vi "MegaVIEW_v_0_0_2.vi"() -> ()   [LabVIEW 2016]
uses:
  <vilib>/Platform/TimedLoop/XDataNode/timing_clust.ctl
  <vilib>/Platform/TimedLoop/XDataNode/nitl_modes.ctl
  <vilib>/Platform/TimedLoop/XDataNode/wakeup.ctl
  <instrlib>/Lake Shore 425/Public/Data/Field Data (Single Reading).vi
  <vilib>/platform/TimedLoop/XDataNode/XDataNode.xnode
  <instrlib>/Lake Shore 425/Lake Shore 425.lvlib
  <vilib>/Platform/TimedLoop/XDataNode/XDNodeRunTimeDep.lvlib
panel:
  out "Numeric":i32
  in  "Position":dbl
  in  "Y Axis":i32(ring) items=["Time", "Position", "Gaussmeter 1", "Gaussmeter 2", "Gaussmeter 3", "Multimeter", "Temp. Monitor"]
  in  "X Axis":i32(ring) items=["Time", "Position", "Gaussmeter 1", "Gaussmeter 2", "Gaussmeter 3", "Multimeter", "Temp. Monitor"]
  out "XY Graph":cluster{dbl[], dbl[]}[](graph)
  in  "Seconds":dbl
  in  "Minutes":dbl
  in  "Hours":dbl
  out "Gaussmeter 3 Chart":dbl(graph)
  out "Gaussmeter 2 Chart":dbl(graph)
  out "Gaussmeter 1 Chart":dbl(graph)
  in  "Gaussmeter 3":bool
  out "Probe Field \nCompensation On 3":bool
  out "Probe Sensitivity 3":dbl=0.001 format="%^.3e"
  out "Probe Serial Number 3":string
  out "Probe Type  3":u16(ring)=40 items=["High Sensitivity"=40, "High Stability"=41, "Ultra-High Sensitivity"=42, "User Programmable Cable / High Sensitivity Probe"=50, "User Programmable Cable / High Stability Probe"=51, "User Programmable Cable / Ultra-High Sensitivity Probe"=52]
  out "Gaussmeter 3 Error":errorcluster
  in  "VISA Gaussmeter 3":refnum<visa-resource-name>
  in  "Gaussmeter 2":bool
  in  "Gaussmeter 1":bool
  in  "stop":bool
  out "Output File Path":path
  in  "Output Folder Path":path
  out "Output File Name":string
  in  "Period [s]":dbl format="%#_3g"
  out "Probe Field \nCompensation On 2":bool
  out "Probe Sensitivity 2":dbl=0.001 format="%^.3e"
  out "Probe Serial Number 2":string
  out "Probe Type  2":u16(ring)=40 items=["High Sensitivity"=40, "High Stability"=41, "Ultra-High Sensitivity"=42, "User Programmable Cable / High Sensitivity Probe"=50, "User Programmable Cable / High Stability Probe"=51, "User Programmable Cable / Ultra-High Sensitivity Probe"=52]
  out "Probe Field \nCompensation On 1":bool
  out "Probe Sensitivity 1":dbl=0.001 format="%^.3e"
  out "Probe Serial Number 1":string
  out "Probe Type 1":u16(ring)=40 items=["High Sensitivity"=40, "High Stability"=41, "Ultra-High Sensitivity"=42, "User Programmable Cable / High Sensitivity Probe"=50, "User Programmable Cable / High Stability Probe"=51, "User Programmable Cable / Ultra-High Sensitivity Probe"=52]
  out "Gaussmeter 2 Error":errorcluster
  out "Gaussmeter 1 Error":errorcluster
  in  "VISA Gaussmeter 2":refnum<visa-resource-name>
  in  "VISA Gaussmeter 1":refnum<visa-resource-name>
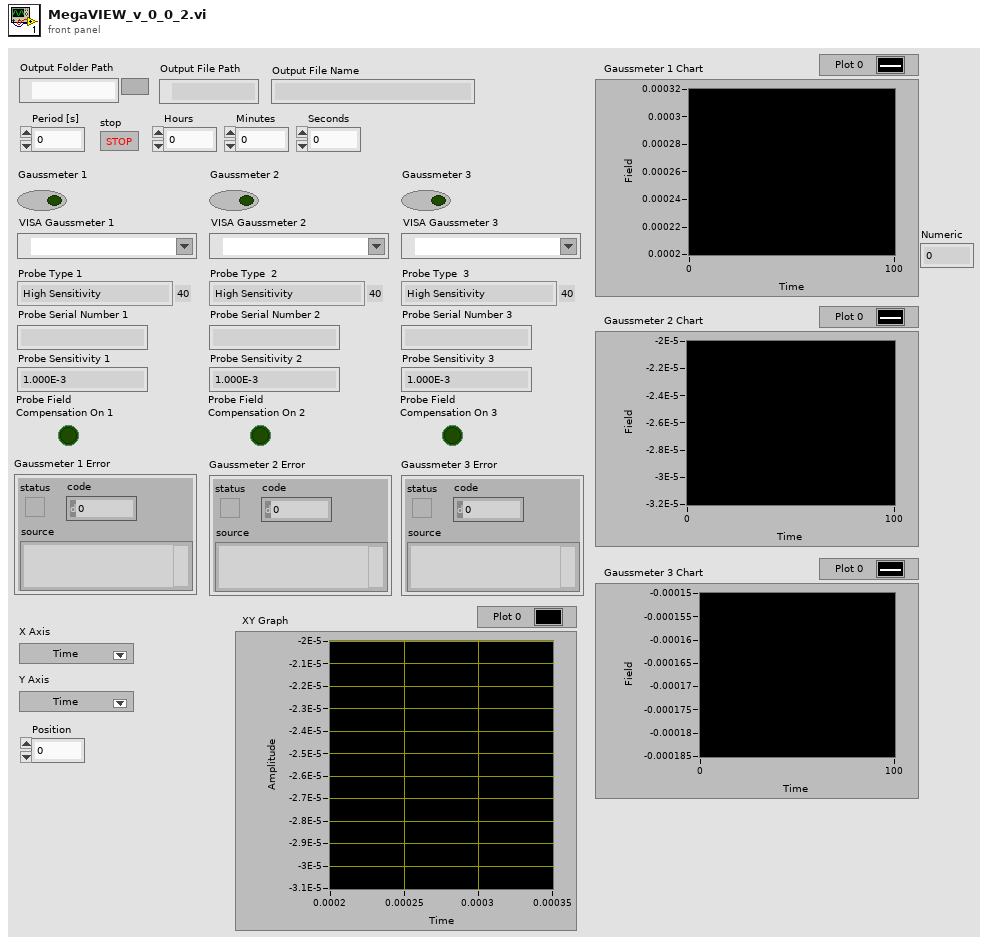
[diagram p1: front panel]
types:
  T1 = enum16{"open", "replace", "create", "open or create", "replace or create", "replace or create with confirmation"}
  T2 = typedef "XDNodeRunTimeDep.lvlib/timing_clust.ctl" = cluster{"Expected End [f-1]":u64, "Actual End [f-1]":u64, "Finished Late? [f-1]":bool, "Expected End [i-1]":u64, "Actual End [i-1]":u64, "Finished Late? [i-1]":bool, "Expected Start [i]":u64, "Actual Start [i]":u64, "Expected Start [f]":u64, "Actual Start [f]":u64, "Source Name":string, "Structure Name":string, "Period":i64, "Deadline":i64, "Offset":i64, "Start":i64, "Priority":i32, "Timeout":i32, "Mode":T3, "Wakeup Reason":T4, "Error":errorcluster, "Source Type":string, "Secondary Source Type":string, "Global End Time":u64, "Global Start Time":u64, "Frame Duration":u64, "Iteration Duration":u64, "Assigned CPU":i32, "I/O Scan Engine Mode":u32}
  T3 = typedef "XDNodeRunTimeDep.lvlib/nitl_modes.ctl" = enum32{"No Change", "Process missed periods, maintain original phase", "Discard missed periods, maintain original phase", "Process missed periods, ignore original phase", "Discard missed periods, ignore original phase"}
  T4 = typedef "XDNodeRunTimeDep.lvlib/wakeup.ctl" = enum32{"Normal", "Aborted", "Asynchronous wakeup", "Timing source error", "Timed loop error", "Timeout"}
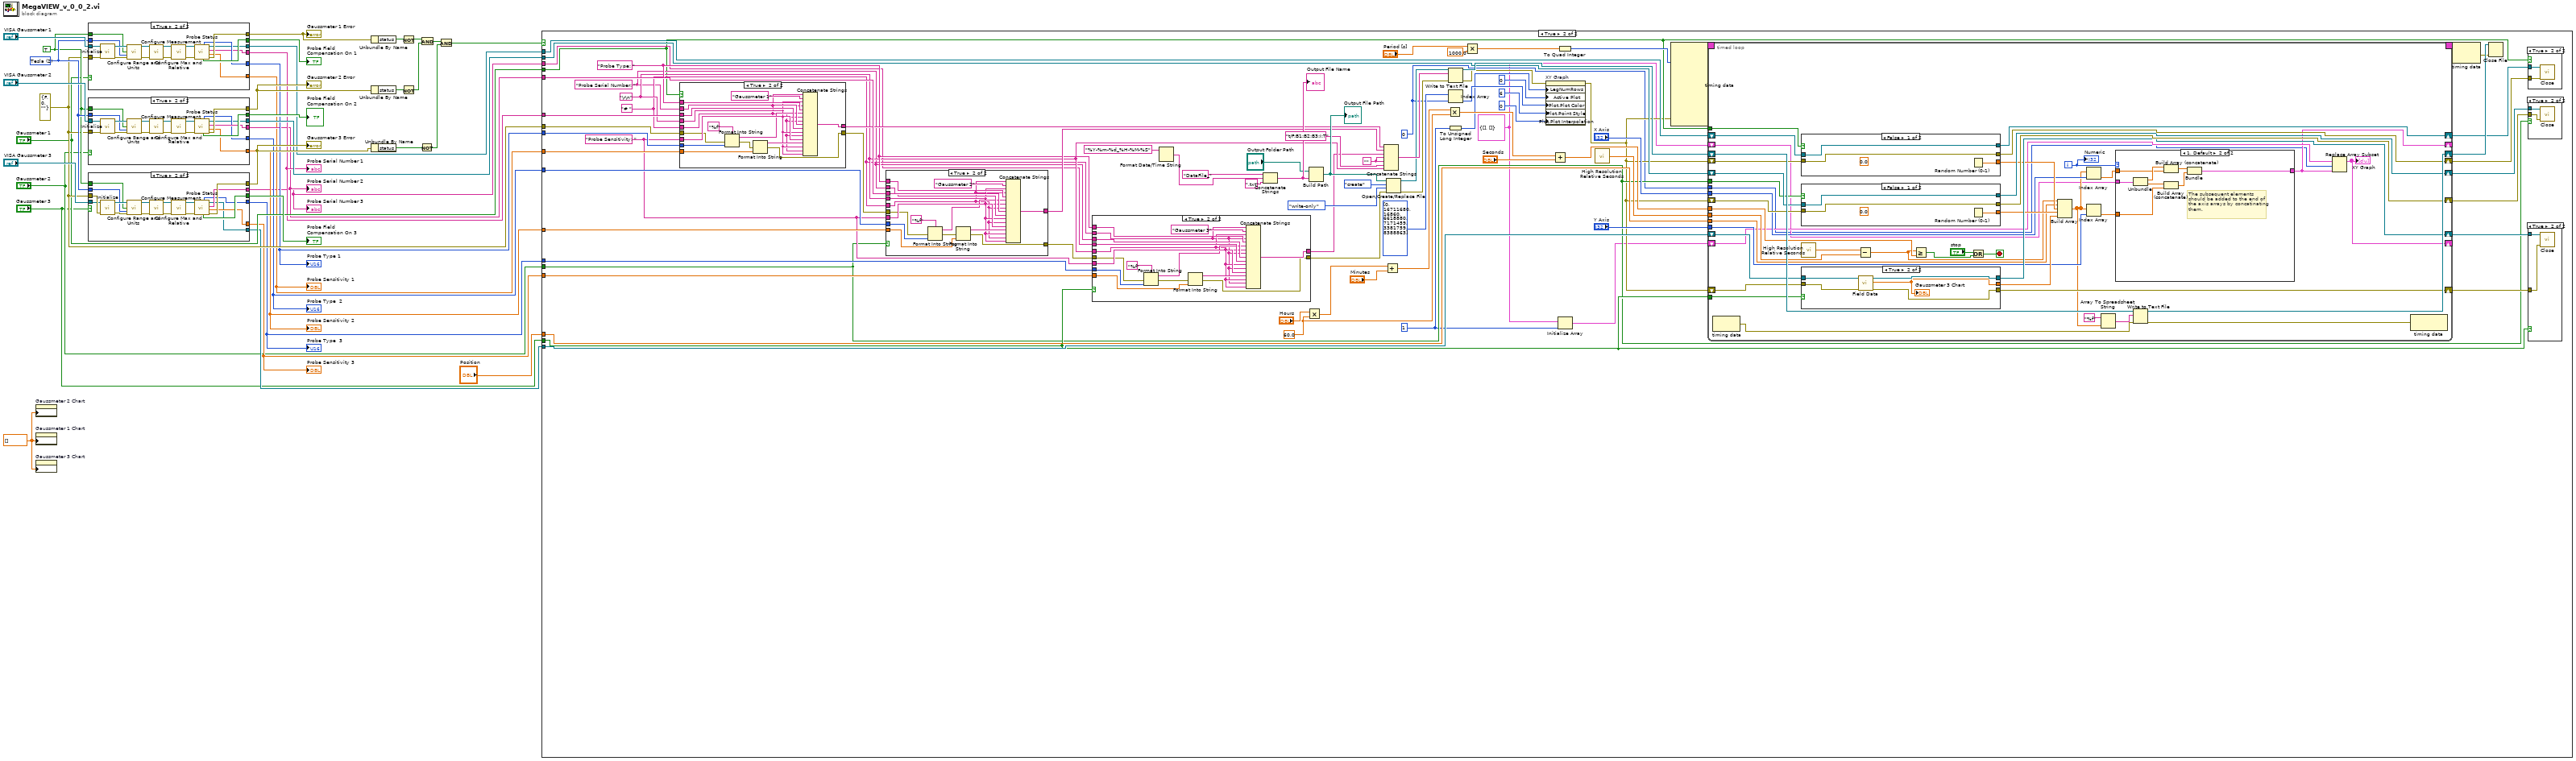
[diagram p0: block diagram]
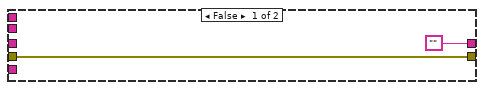
[diagram p6: hidden frame]
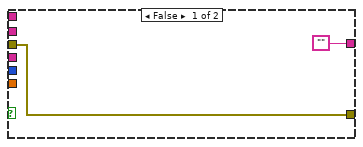
[diagram p7: hidden frame]
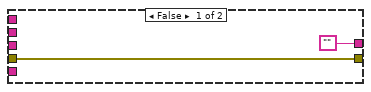
[diagram p8: hidden frame]
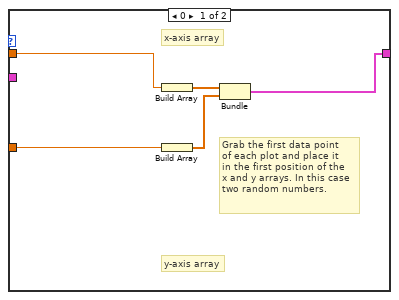
[diagram p9: hidden frame]
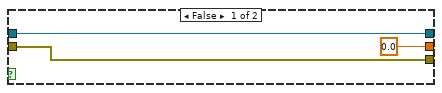
[diagram p10: hidden frame]
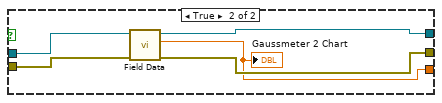
[diagram p11: hidden frame]
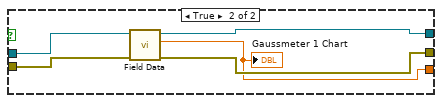
[diagram p12: hidden frame]
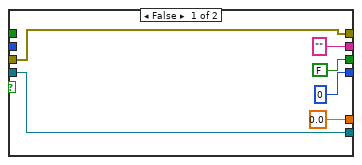
[diagram p13: hidden frame]
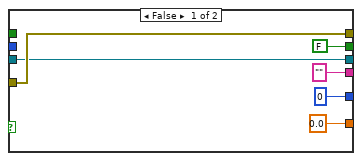
[diagram p14: hidden frame]
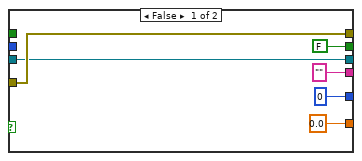
[diagram p15: hidden frame]
diagram:
  w15 = dbl[] [] ("History Data")
  w35 = u16 2 items=["Gauss"=1, "Tesla"=2, "Oersted"=3, "Amp/meter"=4] ("Field Units (1:Gauss)")
  w34 = TRUE ("Auto Range (F: Off)")
  w18 = errorcluster {"status"=FALSE, "code"=0, "source"=""} ("error in (no error)")
  n1 = property on="Gaussmeter 2 Chart" class="WFChart (strict)"("History Data"=w15) -> ()  [unwired: 2 in, 2 out]
  n2 = property on="Gaussmeter 1 Chart" class="WFChart (strict)"("History Data"=w15) -> ()  [unwired: 2 in, 2 out]
  n3 = property on="Gaussmeter 3 Chart" class="WFChart (strict)"("History Data"=w15) -> ()  [unwired: 2 in, 2 out]
  n4 = case shown="True" "Gaussmeter 1" {
    tunnel: "VISA Gaussmeter 1" -> [w38 w61]
    tunnel: w35 -> [_ w58]
    tunnel: w34 -> [_ w57]
    tunnel: w18 -> [w43 w56]
    tunnel: [w43 w55] -> w31
    tunnel: [FALSE w54] -> w19
    tunnel: [u16 0 ("Probe Type") w53] -> w12
    tunnel: ["" ("Probe Serial Number") w52] -> w11
    tunnel: [0.0 ("Probe Sensitivity") w51] -> w8
    tunnel: [w38 w44] -> w16
    frame False {
    }
    frame True {
      n5 = call <instrlib>:"Initialize.vi"("error in (no error)"=w56, "VISA resource name"=w61) -> ("error out"=w59:errorcluster, "VISA resource name out"=w60:refnum<visa-resource-name>)  [unwired: 8 in]
      n6 = call <instrlib>:"Configure Range and Units.vi"("VISA resource name"=w60, "Auto Range (F: Off)"=w57, "Field Units (1:Gauss)"=w58, "error in (no error)"=w59) -> ("VISA resource name out"=w50:refnum<visa-resource-name>, "error out"=w49:errorcluster)  [unwired: 10 in]
      n7 = call <instrlib>:"Configure Measurement.vi"("VISA resource name"=w50, "error in (no error)"=w49) -> ("VISA resource name out"=w46:refnum<visa-resource-name>, "error out"=w47:errorcluster)  [unwired: 12 in]
      n8 = call <instrlib>:"Configure Max and Relative.vi"("VISA resource name"=w46, "error in (no error)"=w47) -> ("VISA resource name out"=w45:refnum<visa-resource-name>, "error out"=w48:errorcluster)  [unwired: 12 in]
      n9 = call <instrlib>:"Probe Status.vi"("error in (no error)"=w48, "VISA resource name"=w45) -> ("error out"=w55:errorcluster, "Probe Sensitivity"=w51:dbl, "Probe Serial Number"=w52:string, "VISA resource name out"=w44:refnum<visa-resource-name>, "Probe Field \nCompensation On"=w54:bool, "Probe Type"=w53:u16)  [unwired: 4 in]
    }
  }
  "Gaussmeter 1 Error" <- w31
  "Probe Field \nCompensation On 1" <- w19
  "Probe Serial Number 1" <- w11
  "Probe Sensitivity 1" <- w8
  "Probe Type 1" <- w12
  n10 = case shown="True" "Gaussmeter 2" {
    tunnel: "VISA Gaussmeter 2" -> [w62 w85]
    tunnel: w35 -> [_ w82]
    tunnel: w34 -> [_ w81]
    tunnel: w18 -> [w67 w80]
    tunnel: [w67 w79] -> w33
    tunnel: [FALSE w78] -> w21
    tunnel: [0.0 ("Probe Sensitivity") w77] -> w9
    tunnel: ["" ("Probe Serial Number") w76] -> w10
    tunnel: [u16 0 ("Probe Type") w75] -> w7
    tunnel: [w62 w68] -> w14
    frame False {
    }
    frame True {
      n11 = call <instrlib>:"Initialize.vi"("error in (no error)"=w80, "VISA resource name"=w85) -> ("error out"=w83:errorcluster, "VISA resource name out"=w84:refnum<visa-resource-name>)  [unwired: 8 in]
      n12 = call <instrlib>:"Configure Range and Units.vi"("VISA resource name"=w84, "Auto Range (F: Off)"=w81, "Field Units (1:Gauss)"=w82, "error in (no error)"=w83) -> ("VISA resource name out"=w71:refnum<visa-resource-name>, "error out"=w72:errorcluster)  [unwired: 10 in]
      n13 = call <instrlib>:"Configure Measurement.vi"("VISA resource name"=w71, "error in (no error)"=w72) -> ("VISA resource name out"=w73:refnum<visa-resource-name>, "error out"=w74:errorcluster)  [unwired: 12 in]
      n14 = call <instrlib>:"Configure Max and Relative.vi"("VISA resource name"=w73, "error in (no error)"=w74) -> ("VISA resource name out"=w70:refnum<visa-resource-name>, "error out"=w69:errorcluster)  [unwired: 12 in]
      n15 = call <instrlib>:"Probe Status.vi"("error in (no error)"=w69, "VISA resource name"=w70) -> ("error out"=w79:errorcluster, "Probe Sensitivity"=w77:dbl, "Probe Serial Number"=w76:string, "VISA resource name out"=w68:refnum<visa-resource-name>, "Probe Field \nCompensation On"=w78:bool, "Probe Type"=w75:u16)  [unwired: 4 in]
    }
  }
  "Gaussmeter 2 Error" <- w33
  "Probe Field \nCompensation On 2" <- w21
  "Probe Sensitivity 2" <- w9
  "Probe Serial Number 2" <- w10
  "Probe Type  2" <- w7
  n16 = case shown="True" "Gaussmeter 3" {
    tunnel: w18 -> [w91 w107]
    tunnel: w35 -> [_ w106]
    tunnel: w34 -> [_ w105]
    tunnel: [w91 w104] -> w32
    tunnel: "VISA Gaussmeter 3" -> [w86 w103]
    tunnel: [FALSE w102] -> w20
    tunnel: [0.0 ("Probe Sensitivity") w101] -> w5
    tunnel: ["" ("Probe Serial Number") w100] -> w4
    tunnel: [u16 0 ("Probe Type") w99] -> w6
    tunnel: [w86 w92] -> w13
    frame False {
    }
    frame True {
      n17 = call <instrlib>:"Initialize.vi"("error in (no error)"=w107, "VISA resource name"=w103) -> ("error out"=w108:errorcluster, "VISA resource name out"=w109:refnum<visa-resource-name>)  [unwired: 8 in]
      n18 = call <instrlib>:"Configure Range and Units.vi"("VISA resource name"=w109, "Auto Range (F: Off)"=w105, "Field Units (1:Gauss)"=w106, "error in (no error)"=w108) -> ("VISA resource name out"=w94:refnum<visa-resource-name>, "error out"=w93:errorcluster)  [unwired: 10 in]
      n19 = call <instrlib>:"Configure Measurement.vi"("VISA resource name"=w94, "error in (no error)"=w93) -> ("VISA resource name out"=w97:refnum<visa-resource-name>, "error out"=w98:errorcluster)  [unwired: 12 in]
      n20 = call <instrlib>:"Configure Max and Relative.vi"("VISA resource name"=w97, "error in (no error)"=w98) -> ("VISA resource name out"=w95:refnum<visa-resource-name>, "error out"=w96:errorcluster)  [unwired: 12 in]
      n21 = call <instrlib>:"Probe Status.vi"("error in (no error)"=w96, "VISA resource name"=w95) -> ("error out"=w104:errorcluster, "Probe Sensitivity"=w101:dbl, "Probe Serial Number"=w100:string, "VISA resource name out"=w92:refnum<visa-resource-name>, "Probe Field \nCompensation On"=w102:bool, "Probe Type"=w99:u16)  [unwired: 4 in]
    }
  }
  "Gaussmeter 3 Error" <- w32
  "Probe Type  3" <- w6
  "Probe Serial Number 3" <- w4
  "Probe Sensitivity 3" <- w5
  "Probe Field \nCompensation On 3" <- w20
  n22 = Unbundle By Name(w31) -> ("status"=w27:bool)
  n23 = Unbundle By Name(w33) -> ("status"=w25:bool)
  n24 = Unbundle By Name(w32) -> ("status"=w24:bool)
  n25 = Not(x=w27) -> (.not. x?=w28:bool)
  n26 = Not(x=w25) -> (.not. x?=w26:bool)
  n27 = Not(x=w24) -> (.not. x?=w23:bool)
  n28 = And(x=w28, y=w26) -> (x .and. y?=w29:bool)
  n29 = And(x=w29, y=w23) -> (x .and. y?=w30:bool)
  n30 = case shown="True" w30 {
    tunnel: w18 -> [_ w136]
    tunnel: "Gaussmeter 1" -> [_ w122]
    tunnel: w16 -> [_ w168]
    tunnel: w14 -> [_ w159]
    tunnel: w13 -> [_ w158]
    tunnel: "Gaussmeter 2" -> [_ w123]
    tunnel: w12 -> [_ w157]
    tunnel: w11 -> [_ w156]
    tunnel: w8 -> [_ w155]
    tunnel: w10 -> [_ w154]
    tunnel: w9 -> [_ w153]
    tunnel: w7 -> [_ w152]
    tunnel: w6 -> [_ w147]
    tunnel: w5 -> [_ w146]
    tunnel: w4 -> [_ w141]
    tunnel: "Gaussmeter 3" -> [_ w124]
    tunnel: "Position" -> [_ w127]
    frame False {
    }
    frame True {
      w111 = 0 ("index")
      w119 = 1 ("dimension size")
      w110 = cluster{dbl[], dbl[]} {[], []}
      w132 = 60.0
      w149 = ""
      w143 = "Probe Serial Number: "
      w142 = "Probe Sensitivity: "
      w148 = "Probe Type: "
      w145 = "\r\n"
      w144 = "# "
      n31 = case shown="True" w122 {
        tunnel: w145 -> [_ w235]
        tunnel: w144 -> [_ w234]
        tunnel: w148 -> [_ w239]
        tunnel: w157 -> [_ w244]
        tunnel: ["" w248] -> w150
        tunnel: w143 -> [_ w247]
        tunnel: w156 -> [_ w246]
        tunnel: w142 -> [_ w245]
        tunnel: w155 -> [_ w241]
        tunnel: [w232 w238] -> w137
        tunnel: w136 -> [w232 w236]
        frame False {
        }
        frame True {
          n32 = Format Into String(format string="%f", error in=w236, w244) -> (resulting string=w243:string, error out=w237:errorcluster)  [unwired: 1 in]
          n33 = Format Into String(error in=w237, w241) -> (resulting string=w240:string, error out=w238:errorcluster)  [unwired: 2 in]
          n34 = Concatenate Strings(w234, "Gaussmeter 1", w235, w234, w239, w243, w235, w234, w247, w246, w235, w234, w245, w240, w235, w234, w235) -> (w248:string)
        }
      }
      n35 = case shown="True" w123 {
        tunnel: w145 -> [_ w217]
        tunnel: w144 -> [_ w216]
        tunnel: w152 -> [_ w226]
        tunnel: ["" w230] -> w151
        tunnel: w143 -> [_ w229]
        tunnel: w154 -> [_ w228]
        tunnel: w142 -> [_ w227]
        tunnel: w153 -> [_ w223]
        tunnel: w148 -> [_ w221]
        tunnel: [w214 w220] -> w138
        tunnel: w137 -> [w214 w218]
        frame False {
        }
        frame True {
          n36 = Format Into String(format string="%f", error in=w218, w226) -> (resulting string=w225:string, error out=w219:errorcluster)  [unwired: 1 in]
          n37 = Format Into String(error in=w219, w223) -> (resulting string=w222:string, error out=w220:errorcluster)  [unwired: 2 in]
          n38 = Concatenate Strings(w216, "Gaussmeter 2", w217, w216, w221, w225, w217, w216, w229, w228, w217, w216, w227, w222, w217, w216, w217) -> (w230:string)
        }
      }
      n39 = case shown="True" w124 {
        tunnel: w145 -> [_ w199]
        tunnel: w144 -> [_ w198]
        tunnel: w147 -> [_ w208]
        tunnel: ["" w212] -> w140
        tunnel: w143 -> [_ w211]
        tunnel: w141 -> [_ w210]
        tunnel: w142 -> [_ w209]
        tunnel: w146 -> [_ w205]
        tunnel: w148 -> [_ w203]
        tunnel: [w196 w202] -> w139
        tunnel: w138 -> [w196 w200]
        frame False {
        }
        frame True {
          n40 = Format Into String(format string="%f", error in=w200, w208) -> (resulting string=w207:string, error out=w201:errorcluster)  [unwired: 1 in]
          n41 = Format Into String(error in=w201, w205) -> (resulting string=w204:string, error out=w202:errorcluster)  [unwired: 2 in]
          n42 = Concatenate Strings(w198, "Gaussmeter 3", w199, w198, w203, w207, w199, w198, w211, w210, w199, w198, w209, w204, w199, w198, w199) -> (w212:string)
        }
      }
      n43 = Format Date/Time String(time format string (%c)="%Y-%m-%d_%H-%M-%S") -> (date/time string=w170:string)  [unwired: 2 in]
      n44 = Concatenate Strings("DataFile_" ("string"), w170, ".txt" ("string")) -> (w180:string)
      "Output File Name" <- w180
      n45 = Multiply(x="Hours", y=w132) -> (x*y=w133:dbl)
      n46 = Build Path(base path="Output Folder Path", name or relative path=w180) -> (appended path=w181:path)
      "Output File Path" <- w181
      n47 = Concatenate Strings(w150, w151, w140, w149, w149, "t/F:B1:B2:B3:I:T", w145) -> (w183:string)
      n48 = Add(x=w133, y="Minutes") -> (x+y=w131:dbl)
      n49 = Open/Create/Replace File(file path (use dialog)=w181, error in=w139, operation (0:open)=T1."create", access (0:read/write)=enum16{"read/write", "read-only", "write-only"}."write-only") -> (refnum out=w182:refnum<file>, error out=w184:errorcluster)  [unwired: 2 in, 1 out]
      n50 = Multiply(x=w131, y=w132) -> (x*y=w135:dbl)
      n51 = To Unsigned Long Integer(number=w119) -> (unsigned 32bit integer=w117:u32)
      n52 = Write to Text File(file (use dialog)=w182, text=w183, error in=w184) -> (refnum out=w186:refnum<file>, error out=w121:errorcluster)  [unwired: 1 in, 1 out]
      n53 = Index Array(array=u32[] [0, 16711680, 16860, 6618880, 7171459, 3381759, 8388863], index=w111) -> (element=w118:u32)
      n54 = Multiply(x="Period [s]", y=1000.0) -> (x*y=w177:dbl)
      n55 = property on="XY Graph" class="XYGraph (strict)"(error in=w121, "LegNumRows"=w117, "Active Plot"=u32 0, "Plot.Plot Color"=w118, "Plot.Point Style"=u8 6, "Plot.Plot Interpolation"=u8 0) -> (error out=w115:errorcluster)  [unwired: 1 in, 1 out]
      n56 = Add(x=w135, y="Seconds") -> (x+y=w128:dbl)
      n57 = To Quad Integer(1:w177) -> (0:w178:i64)
      n58 = Initialize Array(w110, w119) -> (w112:cluster{dbl[], dbl[]}[])
      n59 = call <vilib>:"High Resolution Relative Seconds.vi"() -> ("relative seconds"=w164:dbl)
      n60 = node-c288(w178, w115) -> (w189:T2)  [unwired: 8 in]
      n61 = timed-loop {
        timing: w189 -> [_]
        timing-out: [_] -> w188
        shift-right: [w291] -> w187
        shift-left: w186 -> [w292]
        tunnel: w122 -> [w286]
        shift-right: [w283] -> w166
        shift-left: w115 -> [w282]
        tunnel: w164 -> [w280]
        shift-right: [w278] -> w161
        shift-left: w115 -> [w279]
        shift-right: [w276] -> w162
        shift-left: w115 -> [w274]
        tunnel: w123 -> [w268]
        tunnel: w124 -> [w267]
        shift-right: [w284] -> w167
        shift-left: w168 -> [w285]
        shift-right: [w275] -> w160
        shift-left: w159 -> [w273]
        shift-right: [w277] -> w163
        shift-left: w158 -> [w272]
        tunnel: w128 -> [w264]
        tunnel: w127 -> [w261]
        tunnel: "X Axis" -> [w260]
        tunnel: "Y Axis" -> [w259]
        shift-right: [w257] -> _
        shift-left: w112 -> [w253]
        shift-right: [w251] -> _
        shift-left: w110 -> [w252]
        tunnel: w111 -> [w250]
        i -> [w256]
        stop <- w265 stop-if-true
        n62 = node-c288() -> (w290:errorcluster)  [unwired: 1 in]
        n63 = case shown="False" w286 {
          tunnel: w285 -> [w324 w329]
          tunnel: [w324 w328] -> w284
          tunnel: [w323 w327] -> w283
          tunnel: w282 -> [w323 w326]
          tunnel: [w322 w325] -> w271
          frame False {
            (unwired) 0.0
            n64 = Random Number (0-1)() -> (number: 0 to 1=w322:dbl)
          }
          frame True {
            n65 = call-poly <instrlib>:"Field Data.vi"("error in (no error)"=w326, "VISA resource name"=w329) -> ("error out"=w327:errorcluster, "Field Reading"=w325:dbl, "VISA resource name out"=w328:refnum<visa-resource-name>)  [unwired: 7 in]
            "Gaussmeter 1 Chart" <- w325
          }
        }
        n66 = case shown="False" w268 {
          tunnel: w273 -> [w316 w321]
          tunnel: [w316 w320] -> w275
          tunnel: [w315 w319] -> w278
          tunnel: w279 -> [w315 w318]
          tunnel: [w314 w317] -> w270
          frame False {
            (unwired) 0.0
            n67 = Random Number (0-1)() -> (number: 0 to 1=w314:dbl)
          }
          frame True {
            n68 = call-poly <instrlib>:"Field Data.vi"("error in (no error)"=w318, "VISA resource name"=w321) -> ("error out"=w319:errorcluster, "Field Reading"=w317:dbl, "VISA resource name out"=w320:refnum<visa-resource-name>)  [unwired: 7 in]
            "Gaussmeter 2 Chart" <- w317
          }
        }
        n69 = call <vilib>:"High Resolution Relative Seconds.vi"() -> ("relative seconds"=w281:dbl)
        n70 = case shown="True" w267 {
          tunnel: w272 -> [w308 w313]
          tunnel: [w308 w312] -> w277
          tunnel: [w307 w311] -> w276
          tunnel: w274 -> [w307 w310]
          tunnel: [0.0 w309] -> w269
          frame False {
          }
          frame True {
            n71 = call-poly <instrlib>:"Field Data.vi"("error in (no error)"=w310, "VISA resource name"=w313) -> ("error out"=w311:errorcluster, "Field Reading"=w309:dbl, "VISA resource name out"=w312:refnum<visa-resource-name>)  [unwired: 7 in]
            "Gaussmeter 3 Chart" <- w309
          }
        }
        n72 = Subtract(x=w281, y=w280) -> (x-y=w262:dbl)
        n73 = Greater Or Equal?(x=w262, y=w264) -> (x >= y?=w263:bool)
        n74 = Or(x="stop", y=w263) -> (x .or. y?=w265:bool)
        n75 = Build Array(w262, w261, w271, w270, w269) -> (w258:dbl[])
        n76 = Index Array(array=w258, index=w260) -> (element=w254:dbl)
        n77 = Index Array(array=w258, index=w259) -> (element=w255:dbl)
        n78 = Array To Spreadsheet String(array=w258, 3:"%f" ("format string")) -> (spreadsheet string=w287:string)  [unwired: 1 in]
        n79 = case shown="1, Default" w256 {
          tunnel: [w295 w302] -> w251
          tunnel: w252 -> [_ w298]
          tunnel: w255 -> [w293 w300]
          tunnel: w254 -> [w294 w299]
          frame 0 {
            # "y-axis array"
            # "x-axis array"
            # "Grab the first data point\nof each plot and place it\nin the first position of the \nx and y arrays. In this case\ntwo random numbers."
            n80 = Build Array(w294) -> (w297:dbl[])
            n81 = Build Array(w293) -> (w296:dbl[])
            n82 = Bundle(w297, w296) -> (w295:cluster{dbl[], dbl[]})  [unwired: 1 in]
          }
          frame 1, Default {
            # "The subsequent elements\nshould be added to the end of\nthe axis arrays by concatinating\nthem."
            n83 = Unbundle(w298) -> (w305:dbl[], w301:dbl[])
            n84 = Build Array (concatenate)(w305, w299) -> (w304:dbl[])
            n85 = Build Array (concatenate)(w301, w300) -> (w303:dbl[])
            n86 = Bundle(w304, w303) -> (w302:cluster{dbl[], dbl[]})  [unwired: 1 in]
          }
        }
        n87 = Write to Text File(file (use dialog)=w292, text=w287, error in=w290) -> (refnum out=w291:refnum<file>, error out=w289:errorcluster)  [unwired: 1 in, 1 out]
        n88 = Replace Array Subset(array=w253, new element=w251, index=w250) -> (w257:cluster{dbl[], dbl[]}[])
        "XY Graph" <- w257
        n89 = node-c288(w289) -> ()  [unwired: 1 out]
        "Numeric" <- w256
      }
      n90 = node-c288(w188) -> (w185:errorcluster)
      n91 = Close File(refnum=w187, error in=w185) -> ()  [unwired: 2 out]
      n92 = case shown="True" w122 {
        tunnel: w167 -> [_ w195]
        tunnel: w166 -> [_ w194]
        frame False {
        }
        frame True {
          n93 = call <instrlib>:"Close.vi"("error in (no error)"=w194, "VISA resource name"=w195) -> ()  [unwired: 9 in, 1 out]
        }
      }
      n94 = case shown="True" w123 {
        tunnel: w161 -> [_ w193]
        tunnel: w160 -> [_ w192]
        frame False {
        }
        frame True {
          n95 = call <instrlib>:"Close.vi"("error in (no error)"=w193, "VISA resource name"=w192) -> ()  [unwired: 9 in, 1 out]
        }
      }
      n96 = case shown="True" w124 {
        tunnel: w163 -> [_ w191]
        tunnel: w162 -> [_ w190]
        frame False {
        }
        frame True {
          n97 = call <instrlib>:"Close.vi"("error in (no error)"=w190, "VISA resource name"=w191) -> ()  [unwired: 9 in, 1 out]
        }
      }
    }
  }
